vi "Disconnect.vi"(8 "error in":errorcluster, 11 "TC01 in":refnum<class "TC01.lvclass">) -> (0 "error out":errorcluster, 3 "TC01 out":refnum<class "TC01.lvclass">)   [LabVIEW 2018, in "TC01.lvlib" / "TC01.lvclass"]
uses:
  TC01.lvclass
  TC01.lvclass/TC01.ctl
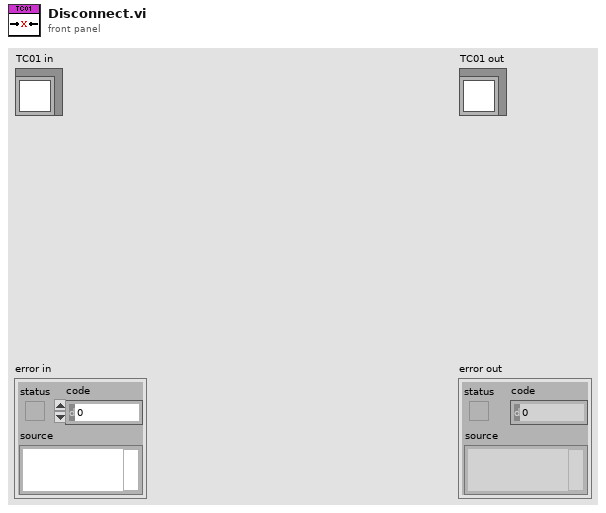
[diagram p1: front panel]
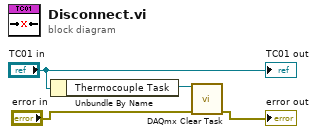
[diagram p0: block diagram]
diagram:
  n1 = Unbundle By Name("TC01 in") -> ("Thermocouple Task"=w4:refnum<k21>)
  n2 = call <vilib>:"DAQmx Clear Task.vi"("task in"=w4, "error in"="error in") -> ("error out"=→"error out":errorcluster)  [unwired: 13 in]
  "TC01 out" <- "TC01 in"
